vi "Helium4 Corrected Pressure.vi"(9 "Tube Radius (mm)":dbl=1.2192, 10 "Warm Temperature (K)":dbl=295.0, 11 "He4 Pressure (mbar)":dbl=0.4 format="%_5e") -> (2 "Corrected He4 Temperature (K)":dbl=0.4 format="%_5e", 3 "Corrected He4 Pressure (mbar)":dbl=0.4 format="%_5e")   [LabVIEW 2020]
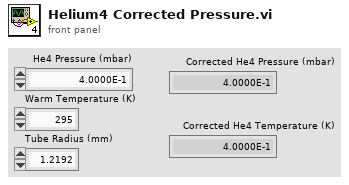
[diagram p1: front panel]
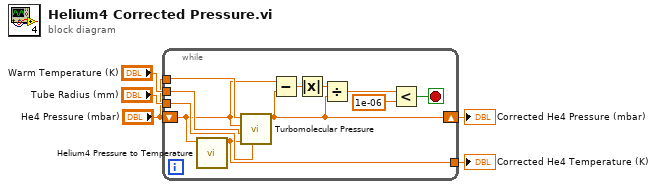
[diagram p0: block diagram]
diagram:
  n1 = while {
    shift-right: [w10] -> w5
    shift-left: "He4 Pressure (mbar)" -> [w11]
    tunnel: "Tube Radius (mm)" -> [w14]
    tunnel: "Warm Temperature (K)" -> [w15]
    tunnel: "He4 Pressure (mbar)" -> [w16]
    tunnel: [w6] -> w1
    stop <- w7 stop-if-true
    n2 = call "Helium4 Pressure to Temperature.vi"("He4 Pressure (mbar)"=w11) -> ("He4 Temperature (K)"=w6:dbl)  [unwired: 10 in]
    n3 = call "Turbomolecular Pressure.vi"("Tube Radius (mm)"=w14, "Temperature Cold (K)"=w6, "Temperature Warm (K)"=w15, "Pressure Cold (mbar)"=w11, "Pressure Warm (mbar)"=w16) -> ("Pressure Function"=w10:dbl)  [unwired: 6 in]
    n4 = Subtract(x=w11, y=w10) -> (x-y=w13:dbl)
    n5 = Absolute Value(x=w13) -> (abs(x)=w12:dbl)
    n6 = Divide(x=w12, y=w10) -> (x/y=w9:dbl)
    n7 = Less?(x=w9, y=1e-06) -> (x < y?=w7:bool)
  }
  "Corrected He4 Pressure (mbar)" <- w5
  "Corrected He4 Temperature (K)" <- w1
